vi "Init.vi"(8 "error in (no error)":errorcluster, 9 "Constant Action Data":string, 10 "HAL GOOP4.lvlib:Instrument Base":refnum<class "Instr Base.lvclass">, 11 "Virt Voltage Generator in":refnum<class "Virt Voltage Generator.lvclass">) -> (0 "error out":errorcluster, 3 "Virt Voltage Generator out":refnum<class "Virt Voltage Generator.lvclass">)   [LabVIEW 2023, in "Virt FGens.lvlib" / "Virt Voltage Generator.lvclass"]
uses:
  Virt Voltage Generator.lvclass
  Virt Voltage Generator.lvclass/Virt Voltage Generator.ctl
  Virt Instrument Base/Virt Instr Base.lvclass
  D:/git/HAL/HAL GOOP4/Virt Instrument Base/Virt Instr Base.lvclass
  D:/git/HAL/HAL GOOP4/FGen/Virtual FGen/Virt Voltage Generator/Virt Voltage Generator.lvclass
  Instrument Base/Instr Base.lvclass
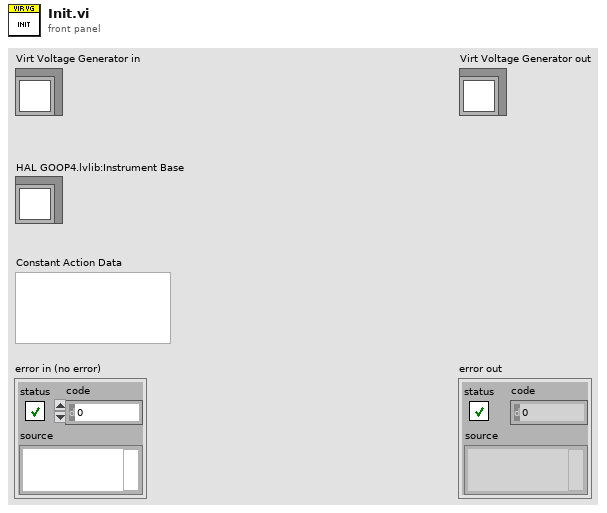
[diagram p1: front panel]
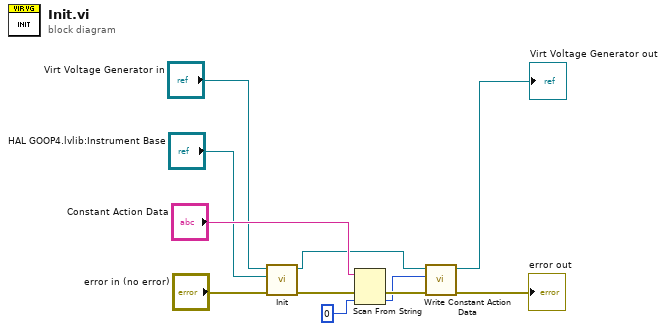
[diagram p0: block diagram]
diagram:
  n1 = call-parent "Init.vi"("error in (no error)"="error in (no error)", "HAL GOOP4.lvlib:Instrument Base"="HAL GOOP4.lvlib:Instrument Base", "Virt Instrument Base in"="Virt Voltage Generator in") -> ("error out"=w5:errorcluster, "Virt Instrument Base out"=w3:refnum<class "Virt Voltage Generator.lvclass">)  [unwired: 7 in]
  n2 = Scan From String(input string="Constant Action Data", error in=w5, default 1=u8 0) -> (error out=w9:errorcluster, output 1=w6:u8)  [unwired: 2 in, 2 out]
  n3 = call "Write Constant Action Data.vi"("error in (no error)"=w9, "Constant Action Data"=w6, "Virt Instrument Base in"=w3) -> ("error out"=→"error out":errorcluster, "Virt Instrument Base in"=→"Virt Voltage Generator out":refnum<class "Virt Voltage Generator.lvclass">)  [unwired: 7 in]
